vi "Split Assignment Statements.vi"(0 "Formulas":string[](array[string])) -> (1 "Assigned Vars":string[](array[string]), 2 "Expressions":string[](array[string]))   [LabVIEW 2020]
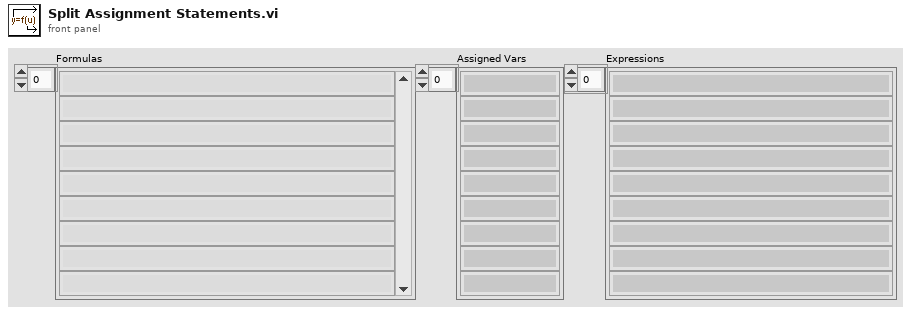
[diagram p1: front panel]
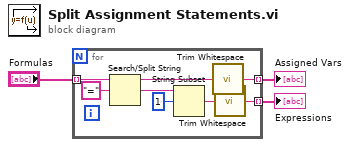
[diagram p0: block diagram]
diagram:
  n1 = for {
    tunnel: "Formulas" -> [w9] mode=indexing
    tunnel: [w5] -> w2 mode=indexing
    tunnel: [w4] -> w1 mode=indexing
    n2 = Search/Split String(string=w9, search string/char (-)="=") -> (substring before match=w8:string, match + rest of string=w11:string)  [unwired: 1 in, 1 out]
    n3 = String Subset(string=w11, offset (0)=1) -> (substring=w7:string)  [unwired: 1 in]
    n4 = call <vilib>:"Trim Whitespace.vi"("string"=w8) -> ("trimmed string"=w5:string)  [unwired: 1 in]
    n5 = call <vilib>:"Trim Whitespace.vi"("string"=w7) -> ("trimmed string"=w4:string)  [unwired: 1 in]
  }
  "Assigned Vars" <- w2
  "Expressions" <- w1
